vi "Main.vi"() -> ()   [LabVIEW 2018]
uses:
  <vilib>/Instr/_visa.llb/VISA Configure Serial Port (Instr).vi
panel:
  out "Input Spectrum":dynamicdata(graph)
  in  "File/DAC":bool
  in  "path":path
  in  "baud rate (9600)":u32=9600
  out "Bytes Written":u32
  in  "VISA resource name":refnum<visa-resource-name>
  in  "stop":bool
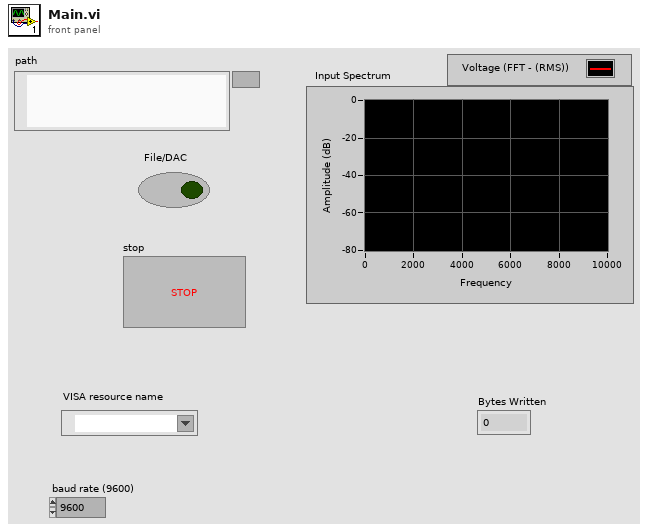
[diagram p1: front panel]
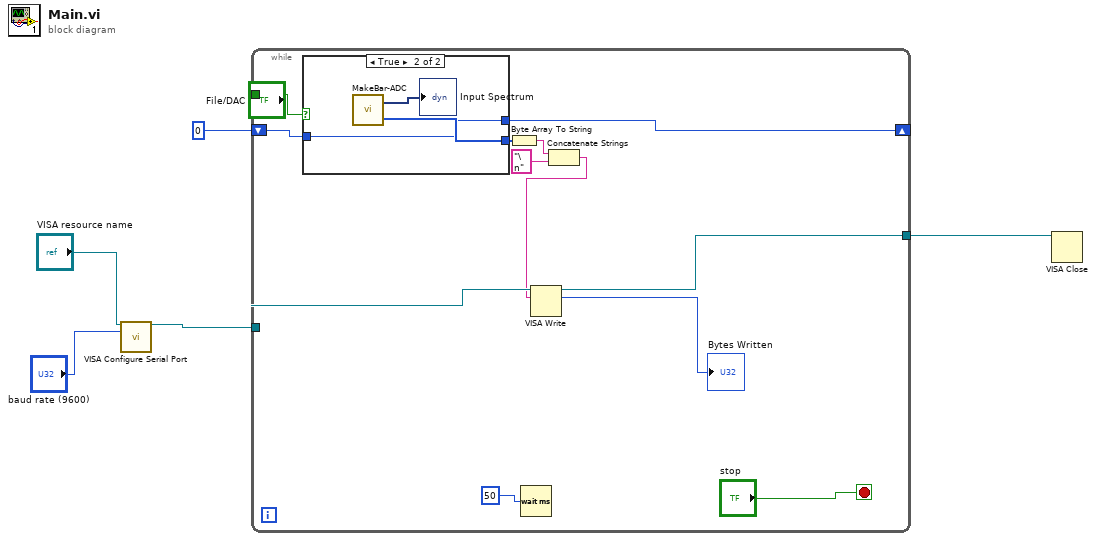
[diagram p0: block diagram]
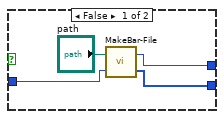
[diagram p2: hidden frame]
diagram:
  n1 = call-poly "VISA Configure Serial Port"("VISA resource name"="VISA resource name", "baud rate (9600)"="baud rate (9600)") -> ("VISA resource name out"=w3:refnum<visa-resource-name>)  [unwired: 12 in, 1 out]
  n2 = while {
    tunnel: [w16] -> w6
    tunnel: w3 -> [w14]
    shift-right: [w12] -> _
    shift-left: 0 ("offset") -> [w11]
    tunnel: "File/DAC" -> [w7]
    stop <- "stop" stop-if-true
    n3 = case shown="True" w7 {
      tunnel: [w22 w25] -> w13
      tunnel: [w20 w24] -> w12
      tunnel: w11 -> [w19 w24]
      frame False {
        n4 = call "MakeBar-File.vi"("position offset"=w19, "path"="path") -> ("output array"=w22:u8[], "offset"=w20:i32)
      }
      frame True {
        n5 = call "MakeBar-ADC.vi"() -> ("output array"=w25:u8[], "Input Spectrum"=→"Input Spectrum":dynamicdata)  [unwired: 2 in]
      }
    }
    n6 = Byte Array To String(unsigned byte array=w13) -> (string=w10:string)
    n7 = Wait (ms)(milliseconds to wait=u32 50) -> ()  [unwired: 1 out]
    n8 = Concatenate Strings(w10, "\n" ("string")) -> (w8:string)
    n9 = VISA Write(VISA resource name=w14, write buffer=w8) -> (VISA resource name out=w16:refnum<visa-resource-name>, return count=→"Bytes Written":u32)  [unwired: 1 in, 1 out]
  }
  n10 = VISA Close(VISA resource name=w6) -> ()  [unwired: 1 in, 1 out]
